vi "DQtoAlphaBeta__src.vi"   [LabVIEW 2017]
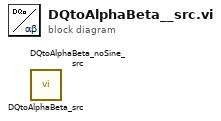
[diagram p0: block diagram]
diagram:
  n1 = call "DQtoAlphaBeta_src.vi"() -> ()  [unwired: 12 in, 4 out]
  n2 = call "DQtoAlphaBeta_noSine_src.vi"() -> ()  [unwired: 14 in, 2 out]
